vi "Get Socket Physical Name PDU Digital Input.vi"(8 "error In":errorcluster, 10 "ChannelType":string) -> (0 "error out":errorcluster, 2 "Physical Channel":tag[](array[tag]), 3 "Physical String":string[](array[string]))   [LabVIEW 2023, in "HardwareAbstractionLayer_LVOOP.lvlib" / "Teststand.lvclass"]
doc: "This VI Filter Physical Channel and Number Socket Running"
uses:
  Teststand.lvclass
  Database/Database.lvclass
panel:
  in  "Number Of DUT":i32
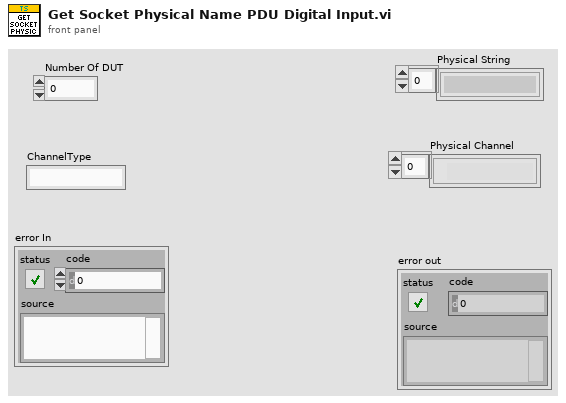
[diagram p1: front panel]
types:
  T1 = typedef "HardwareAbstractionLayer_LVOOP.lvlib/Teststand.lvclass/Teststand Status Control.ctl" = cluster{"Terminating or Aborting":bool, "Stop":bool, "Socket Count":i16, "Selected Sockets":i16[]}
  T2 = cluster{"table":string, "condition":string, "columns":string[]}
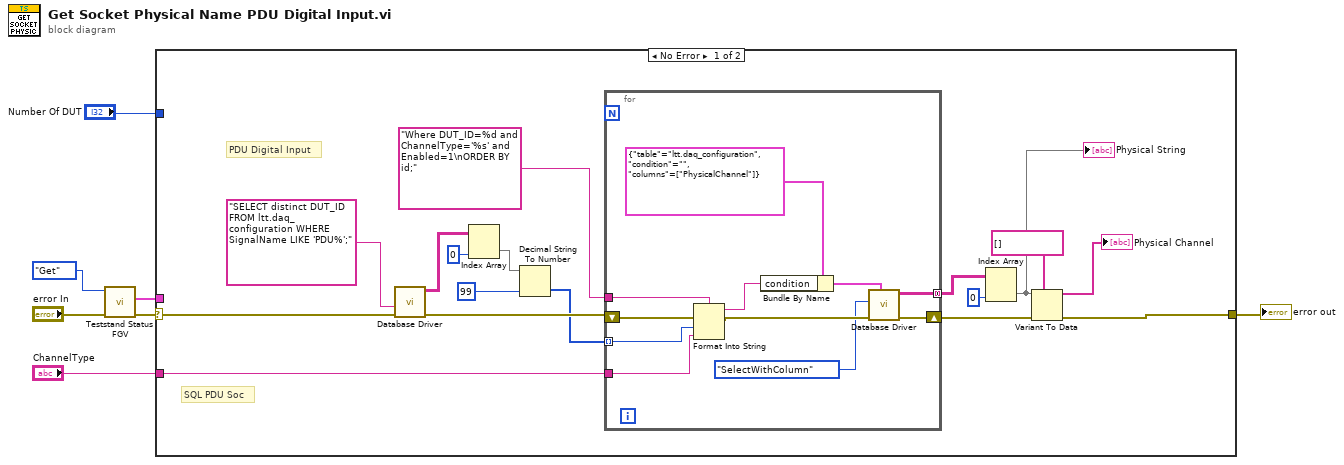
[diagram p0: block diagram]
diagram:
  n1 = call "Teststand Status FGV.vi"("error in"="error In", "Option"=enum16{"Set", "Get"}."Get") -> ("error out"=w3:errorcluster, "Teststand Status Out"=w2:T1)  [unwired: 8 in]
  n2 = case shown="No Error" w3 {
    selector: w3 -> [w10 w36]
    tunnel: "ChannelType" -> [w17 _]
    tunnel: [w16 w36] -> w6
    tunnel: w2 -> [_ _]
    tunnel: "Number Of DUT" -> [_ _]
    frame No Error {
      # "PDU Digital Input"
      # "SQL PDU Soc"
      n3 = call "Database Driver.vi"("error in"=w10, "SQL query"="SELECT distinct DUT_ID FROM ltt.daq_configuration WHERE SignalName LIKE 'PDU%';") -> ("error out"=w9:errorcluster, "data"=w14:string[][])  [unwired: 6 in, 2 out]
      n4 = Index Array(array=w14, index (col)=0 ("disabled index (col)")) -> (element=w15:string[])  [unwired: 1 in]
      n5 = Decimal String To Number(string=w15, default (0L)=i16 99 ("Numeric")) -> (number=w8:i16[])  [unwired: 1 in, 1 out]
      n6 = for {
        tunnel: "Where DUT_ID=%d and ChannelType='%s' and Enabled=1\nORDER BY id;" -> [w35]
        shift-right: [w28] -> w24
        shift-left: w9 -> [w32]
        tunnel: [w27] -> w23 mode=concatenating
        tunnel: w17 -> [w31]
        tunnel: w8 -> [w25] mode=indexing
        n7 = Format Into String(format string=w35, error in=w32, w25, w31) -> (resulting string=w33:string, error out=w29:errorcluster)  [unwired: 1 in]
        n8 = Bundle By Name(cluster=T2 {"table"="ltt.daq_configuration", "condition"="", "columns"=["PhysicalChannel"]} ("SQLTableData"), "condition"=w33) -> (w30:T2)
        n9 = call "Database Driver.vi"("SQLTableData"=w30, "error in"=w29, "Select"=enum16{"SelectWithQuery", "SelectWithColumn"}."SelectWithColumn") -> ("error out"=w28:errorcluster, "data"=w27:string[][])  [unwired: 5 in, 2 out]
      }
      n10 = Index Array(array=w23, index (col)=0 ("disabled index (col)")) -> (element=w22:string[])  [unwired: 1 in]
      "Physical String" <- w22
      n11 = Variant To Data(error in=w24, type=tag[] [] ("AI.PhysicalChans"), Variant=w22) -> (data=→"Physical Channel":tag[], error out=w16:errorcluster)
    }
    frame Error {
    }
  }
  "error out" <- w6
